vi "Convert TDMS to Excel.vi"(8 "error in":errorcluster, 9 "Show Configure Dialog?":bool, 10 "Remove Extra Properties? (T)":bool=TRUE, 11 "Path to TDMS/TDM File":path) -> (0 "error out":errorcluster)   [LabVIEW 2020, in "Logging.lvlib" / "Logging.lvclass"]
doc: "This VI will convert a TDMS file to a XLSX file. Excel 2007, and the TDMS Add on for Excel needs to be installed. Then provide the path to the TDMS or TDM file. A file with the same name in the same directory will be created with a .XLSX file extension.\n\nBy default the conversion will remove many extra properties that aren't always used. To include all properties make \"Remove Extra Properties\" false. If you would like to choose the properties to include set \"Show Configure Dialog\" to be true.\n\nBrian Hoover (hooovahh) 2010"
uses:
  <userlib>/_OpenG.lib/file/file.llb/Strip Path Extension - String__ogtk.vi
  Logging/Logging.lvclass
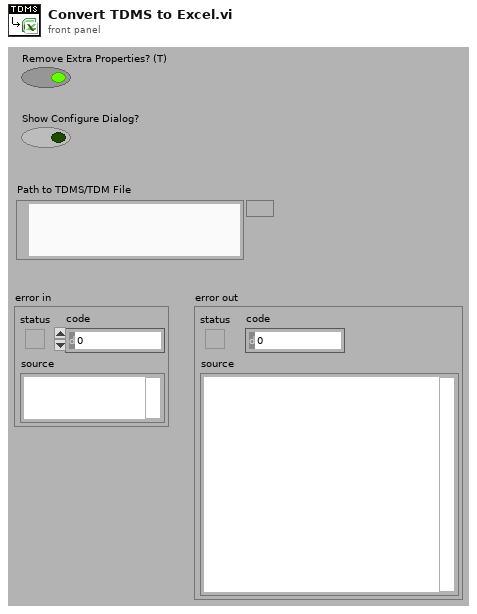
[diagram p1: front panel]
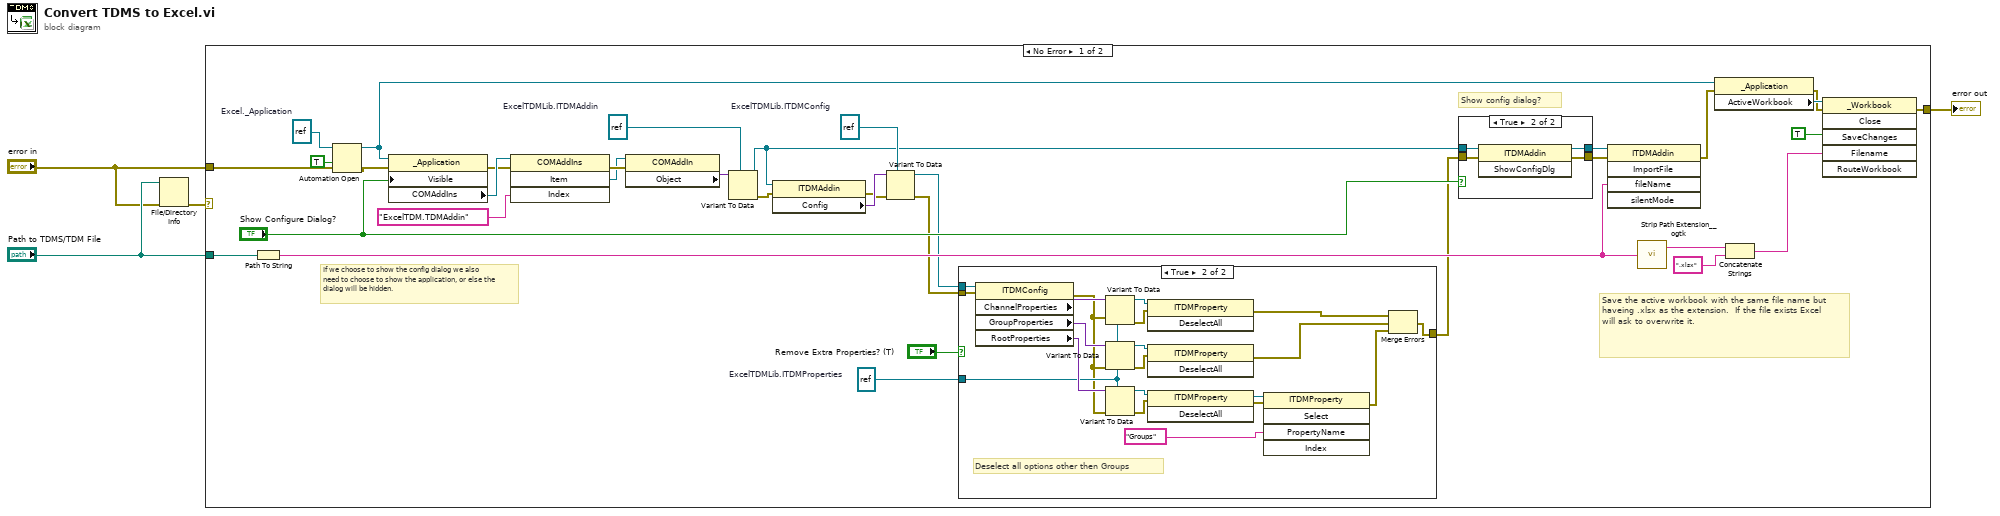
[diagram p0: block diagram]
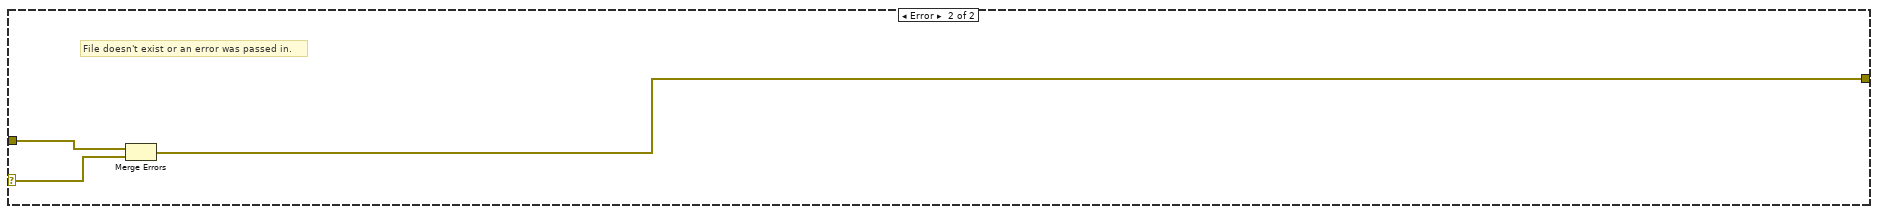
[diagram p4: hidden frame]
diagram:
  n1 = File/Directory Info(path="Path to TDMS/TDM File", error in="error in") -> (error out=w3:errorcluster)  [unwired: 6 out]
  n2 = case shown="No Error" w3 {
    selector: w3 -> [_ w68]
    tunnel: "Path to TDMS/TDM File" -> [w30 _]
    tunnel: [w25 w67] -> w1
    tunnel: "error in" -> [w8 w69]
    frame No Error {
      w9 = refnum<k7> refnum  # Excel._Application
      w18 = refnum<k7> refnum  # ExcelTDMLib.ITDMProperties
      w19 = refnum<k7> refnum  # ExcelTDMLib.ITDMConfig
      w38 = refnum<k7> refnum  # ExcelTDMLib.ITDMAddin
      # "Save the active workbook with the same file name but haveing .xlsx as the extension.  If the file exists Excel will ask to overwrite it."
      # "Show config dialog?"
      # "If we choose to show the config dialog we also need to choose to show the application, or else the dialog will be hidden."
      n3 = Path To String(path=w30) -> (string=w29:string)
      n4 = Automation Open(error in (no error)=w8, Automation Refnum=w9, 9:TRUE ("open new instance (false)")) -> (Automation Refnum=w6:refnum<k7>, error out=w7:errorcluster)  [unwired: 1 in]
      n5 = property class="_Application"(reference=w6, error in=w7, "Visible"="Show Configure Dialog?") -> (error out=w34:errorcluster, "COMAddIns"=w39:refnum<k7>)  [unwired: 1 out]
      n6 = invoke class="COMAddIns" method="Item"(reference=w39, error in=w34, "Index"="ExcelTDM.TDMAddin") -> (error out=w36:errorcluster, "Item"=w35:refnum<k7>)  [unwired: 1 in, 2 out]
      n7 = property class="COMAddIn"(reference=w35, error in=w36) -> ("Object"=w20:variant)  [unwired: 2 out]
      n8 = Variant To Data(type=w38, Variant=w20) -> (data=w17:refnum<k7>, error out=w15:errorcluster)  [unwired: 1 in]
      n9 = property class="ITDMAddin"(reference=w17, error in=w15) -> (error out=w14:errorcluster, "Config"=w16:variant)  [unwired: 1 out]
      n10 = Variant To Data(error in=w14, type=w19, Variant=w16) -> (data=w12:refnum<k7>, error out=w13:errorcluster)
      n11 = case shown="True" "Remove Extra Properties? (T)" {
        tunnel: w18 -> [_ w56]
        tunnel: w13 -> [w40 w47]
        tunnel: w12 -> [_ w46]
        tunnel: [w40 w45] -> w11
        frame False {
        }
        frame True {
          # "Deselect all options other then Groups"
          n12 = property class="ITDMConfig"(reference=w46, error in=w47) -> (error out=w51:errorcluster, "ChannelProperties"=w60:variant, "GroupProperties"=w58:variant, "RootProperties"=w57:variant)  [unwired: 1 out]
          n13 = Variant To Data(error in=w51, type=w56, Variant=w60) -> (data=w59:refnum<k7>, error out=w48:errorcluster)
          n14 = Variant To Data(error in=w51, type=w56, Variant=w58) -> (data=w54:refnum<k7>, error out=w49:errorcluster)
          n15 = Variant To Data(error in=w51, type=w56, Variant=w57) -> (data=w55:refnum<k7>, error out=w50:errorcluster)
          n16 = invoke class="ITDMProperty" method="DeselectAll"(reference=w59, error in=w48) -> (error out=w52:errorcluster)  [unwired: 1 in, 2 out]
          n17 = invoke class="ITDMProperty" method="DeselectAll"(reference=w54, error in=w49) -> (error out=w53:errorcluster)  [unwired: 1 in, 2 out]
          n18 = invoke class="ITDMProperty" method="DeselectAll"(reference=w55, error in=w50) -> (reference out=w44:refnum<k7>, error out=w43:errorcluster)  [unwired: 1 in, 1 out]
          n19 = invoke class="ITDMProperty" method="Select"(reference=w44, error in=w43, "PropertyName"="Groups" ("string")) -> (error out=w42:errorcluster)  [unwired: 2 in, 4 out]
          n20 = Merge Errors(w52, w53, w42) -> (w45:errorcluster)
        }
      }
      n21 = case shown="True" "Show Configure Dialog?" {
        tunnel: w17 -> [w62 w66]
        tunnel: w11 -> [w61 w65]
        tunnel: [w61 w64] -> w23
        tunnel: [w62 w63] -> w22
        frame False {
        }
        frame True {
          n22 = invoke class="ITDMAddin" method="ShowConfigDlg"(reference=w66, error in=w65) -> (reference out=w63:refnum<k7>, error out=w64:errorcluster)  [unwired: 1 in, 1 out]
        }
      }
      n23 = invoke class="ITDMAddin" method="ImportFile"(reference=w22, error in=w23, "fileName"=w29) -> (error out=w33:errorcluster)  [unwired: 2 in, 4 out]
      n24 = call-poly <userlib>:"Strip Path Extension__ogtk.vi"("path"=w29) -> ("root"=w28:string)  [unwired: 1 out]
      n25 = property class="_Application"(reference=w6, error in=w33) -> (error out=w24:errorcluster, "ActiveWorkbook"=w32:refnum<k7>)  [unwired: 1 out]
      n26 = Concatenate Strings(w28, ".xlsx" ("string")) -> (w26:string)
      n27 = invoke class="_Workbook" method="Close"(reference=w32, error in=w24, "SaveChanges"=TRUE, "Filename"=w26) -> (error out=w25:errorcluster)  [unwired: 2 in, 5 out]
    }
    frame Error {
      # "File doesn't exist or an error was passed in."
      n28 = Merge Errors(w69, w68) -> (w67:errorcluster)
    }
  }
  "error out" <- w1
